vi "libssh2_scp_send64.vi"(4 "mtime (0 = current time)":i64, 6 "atime (0 = current time)":i64, 7 "size":i64, 8 "error in (no error)":errorcluster, 9 "mode":i32 format="%.0o", 10 "path":string, 11 "session":T2) -> (0 "error out":errorcluster, 3 "channel":T1)   [LabVIEW 2013, in "libssh2.lvlib"]
doc: "Send a file to an SSH server."
uses:
  libssh2.lvlib
  Session Refnum.ctl
  Channel Refnum.ctl
  Not A Session.vi
  <vilib>/Utility/error.llb/Error Cluster From Error Code.vi
  Global Settings.vi
  Read Session Refnum.vi
  <vilib>/Utility/semaphor.llb/Acquire Semaphore.vi
  <vilib>/Utility/semaphor.llb/Release Semaphore.vi
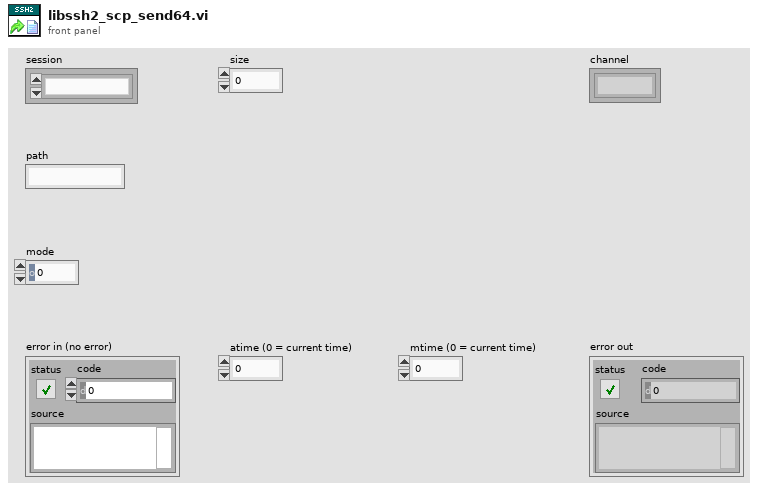
[diagram p1: front panel]
types:
  T1 = typedef "libssh2.lvlib/Channel Refnum.ctl" = refnum<k1>
  T2 = typedef "libssh2.lvlib/Session Refnum.ctl" = refnum<k1>
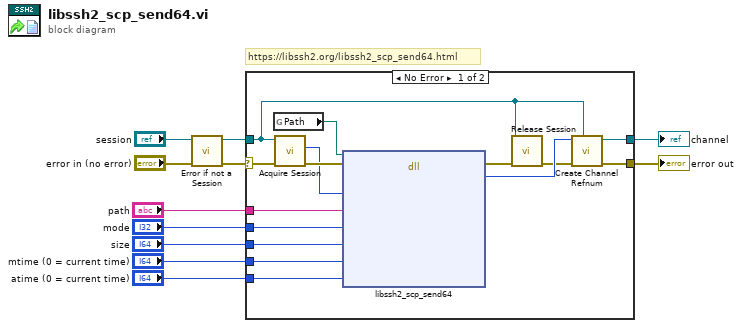
[diagram p0: block diagram]
diagram:
  # "https://libssh2.org/libssh2_scp_send64.html"
  n1 = call "Error if not a Session.vi"("error in (no error)"="error in (no error)", "session"="session") -> ("error out"=w8:errorcluster, "session out"=w6:T2)  [unwired: 8 in]
  n2 = case shown="No Error" w8 {
    selector: w8 -> [w20 w27]
    tunnel: w6 -> [w12 _]
    tunnel: [w23 w27] -> w11
    tunnel: [w21 _] -> w10
    tunnel: "path" -> [w18 _]
    tunnel: "mode" -> [w17 _]
    tunnel: "size" -> [w16 _]
    tunnel: "mtime (0 = current time)" -> [w15 _]
    tunnel: "atime (0 = current time)" -> [w14 _]
    frame No Error {
      n3 = global read "Global Settings.vi" "Path"() -> (w19:path)
      n4 = call "Acquire Session.vi"("error in (no error)"=w20, "session"=w12) -> ("error out"=w25:errorcluster, "LIBSSH2_SESSION*"=w24:u64)  [unwired: 7 in, 1 out]
      n5 = dll-call lib="?" fn="libssh2_scp_send64"(path in=w19, error in=w25, "session"=w24, "path"=w18, "mode"=w17, "size"=w16, "mtime"=w15, "atime"=w14) -> (error out=w26:errorcluster, "return value"=w22:u64)  [unwired: 7 in, 1 out]
      n6 = call "Release Session.vi"("error in (no error)"=w26, "session"=w12) -> ("error out"=w13:errorcluster)  [unwired: 9 in]
      n7 = call "Create Channel Refnum.vi"("session"=w12, "error in (no error)"=w13, "LIBSSH2_CHANNEL*"=w22) -> ("error out"=w23:errorcluster, "channel"=w21:T1)  [unwired: 7 in]
    }
    frame Error {
    }
  }
  "error out" <- w11
  "channel" <- w10
